vi "pump rpm 3-stop.vi"(0 "flow rate":dbl[unit] format="%.2f", 1 "tubing ID":dbl[unit] format="%.2f") -> (3 "pump speed (rpm)":dbl format="%.2f", 5 "in range":bool)   [LabVIEW 2010]
uses:
  Stamp/calibration commands.ctl
panel:
  out "first row":sgl[](array[numeric])=[0.13, 0.19, 0.25, 0.38, 0.44, 0.51, 0.57, 0.64, 0.76, 0.89, 0.95, 1.02, 1.09, 1.14, 1.22, 1.3, 1.42, 1.52, 1.65, 1.75, 1.85, 2.06, 2.29, 2.54, 2.79, 3.17] format="%.3f"
  in  "Ring":u16(ring)
  in  "3-stop tubing":T1(ring)
  # "orange-black\norange-red\norange-blue\norange-green\ngreen-yellow\norange-yellow\nwhite-yellow\norange-white\nblack-black\norange-orange\nwhite-black\nwhite-white\nwhite-red\nred-red\nred-grey\ngrey-grey\nyellow-yellow\nyellow-blue\nblue-blue\nblue-green\ngreen-green\npurple-purple\npurple-black\npurple-orange\npurple-white\nblack-white"
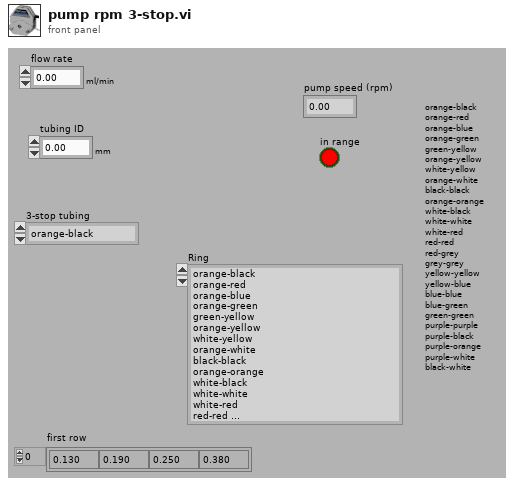
[diagram p1: front panel]
types:
  T1 = enum16{"orange-black", "orange-red", "orange-blue", "orange-green", "green-yellow", "orange-yellow", "white-yellow", "orange-white", "black-black", "orange-orange", "white-black", "white-white", "white-red", "red-red", "red-grey", "grey-grey", "yellow-yellow", "yellow-blue", "blue-blue", "blue-green", "green-green", "purple-purple", "purple-black", "purple-orange", "purple-white", "black-white"}
  T2 = typedef "calibration commands.ctl" = enum16{"Get ini Path", "Save default values", "Save new calibration", "Read calibration", "Apply calibration", "Read STAMP mb", "Write STAMP mb"}
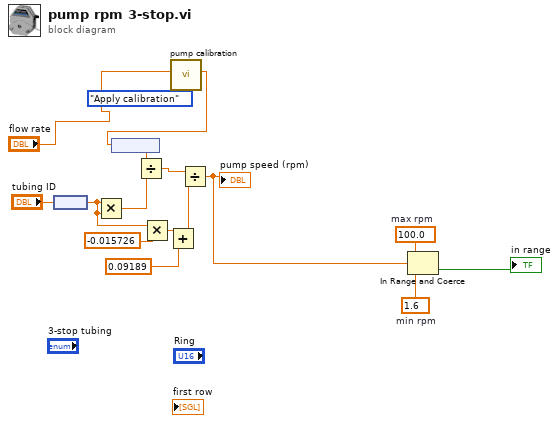
[diagram p0: block diagram]
diagram:
  w8 = 1.6  # min rpm
  w9 = 100.0  # max rpm
  n1 = node("tubing ID") -> (w5:dbl)
  n2 = Multiply(x=w5, y=w5) -> (x*y=w6:dbl)
  n3 = Multiply(x=w5, y=-0.015726) -> (x*y=w12:dbl)
  n4 = Add(x=w12, y=0.09189) -> (x+y=w10:dbl)
  n5 = call "pump calibration.vi"("pump cal command"=calibration_commands."Apply calibration", "flow rate"="flow rate") -> ("modified flow rate"=w1:dbl[unit])  [unwired: 3 in, 3 out]
  n6 = node(w1) -> (w3:dbl)
  n7 = Divide(x=w3, y=w6) -> (x/y=w14:dbl)
  n8 = Divide(x=w14, y=w10) -> (x/y=w7:dbl)
  "pump speed (rpm)" <- w7
  n9 = In Range and Coerce(upper limit=w9, x=w7, lower limit=w8) -> (In Range?=→"in range":bool)  [unwired: 1 out]
